vi "Get EasyXML Data Type.vi"(8 "error in":errorcluster, 10 "LabVIEW Data":variant) -> (0 "error out":errorcluster, 2 "EasyXML Type":T1=enum."Cluster")   [LabVIEW 2013]
uses:
  Type Defs/Formatting Data Type -- Enum.ctl
  <userlib>/_OpenG.lib/lvdata/lvdata.llb/Type Descriptor Enumeration__ogtk.ctl
  JKI Reuse Candidates/Is an Error (error cluster)__JKI Error Handling.vi
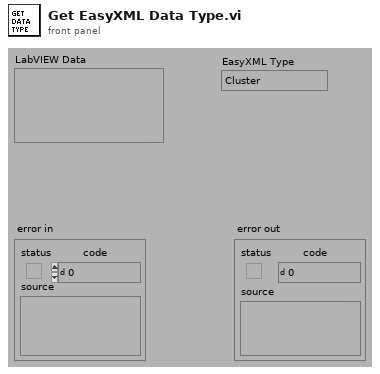
[diagram p1: front panel]
types:
  T1 = typedef "Formatting Data Type -- Enum.ctl" = enum16{"<unknown>", "Cluster", "Array", "String", "Path", "Boolean", "Time Stamp", "Enum", "Numeric - EXT", "Numeric - DBL", "Numeric - SGL", "Numeric - I64", "Numeric - I32", "Numeric - I16", "Numeric - I8", "Numeric - U64", "Numeric - U32", "Numeric - U16", "Numeric - U8", "Numeric - CXT", "Numeric - CDB", "Numeric - CSG", "VISA Resource"}
  T2 = typedef "Type Descriptor Enumeration__ogtk.ctl" = enum8{"<Null>", "I8", "I16", "I32", "I64", "U8", "U16", "U32", "U64", "SGL", "DBL", "EXT", "CSG", "CDB", "CXT", "0x0F", "0x10", "0x11", "0x12", "0x13", "0x14", "Enum U8", "Enum U16", "Enum U32", "Enum U64", "SGL PQ", "DBL PQ", "EXT PQ", "CSG PQ", "CDB PQ", "CXT PQ", "0x1F", "0x20", "Boolean", "0x22", "0x23", "0x24", "0x25", "0x26", "0x27", "0x28", "0x29", "0x2A", "0x2B", "0x2C", "0x2D", "0x2E", "0x2F", "String", "0x31", "Path", "Pict", "0x34", "0x35", "0x36", "DAQ", "0x38", "0x39", "0x3A", "0x3B", "0x3C", "0x3D", "0x3E", "0x3F", "Array", "0x41", "0x42", "0x43", "0x44", "0x45", "0x46", "0x47", "0x48", "0x49", "0x4A", "0x4B", "0x4C", "0x4D", "0x4E", "0x4F", "Cluster", "0x51", "0x52", "Variant", "Waveform", "0x55", "0x56", "0x57", "0x58", "0x59", "0x5A", "0x5B", "0x5C", "0x5D", "0x5E", "0x5F", "0x60", "0x61", "0x62", "0x63", "0x64", "0x65", "0x66", "0x67", "0x68", "0x69", "0x6A", "0x6B", "0x6C", "0x6D", "0x6E", "0x6F", "Refnum"}
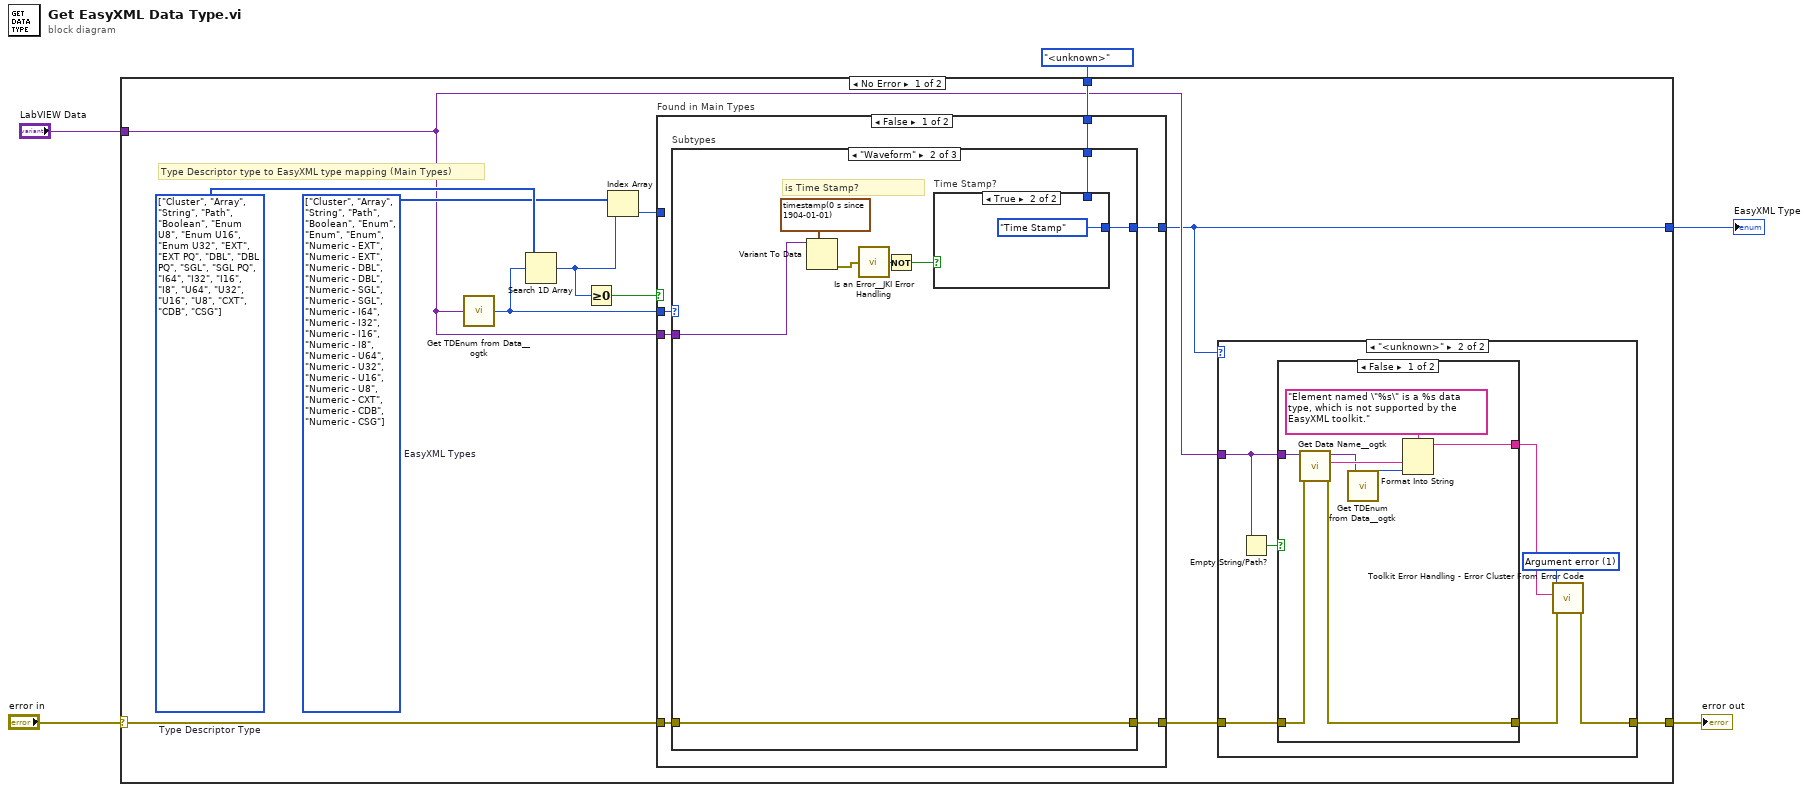
[diagram p0: block diagram]
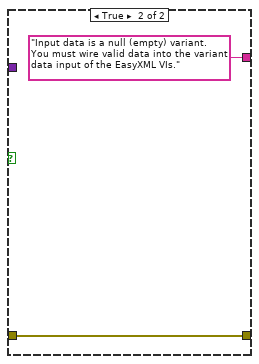
[diagram p3: hidden frame]
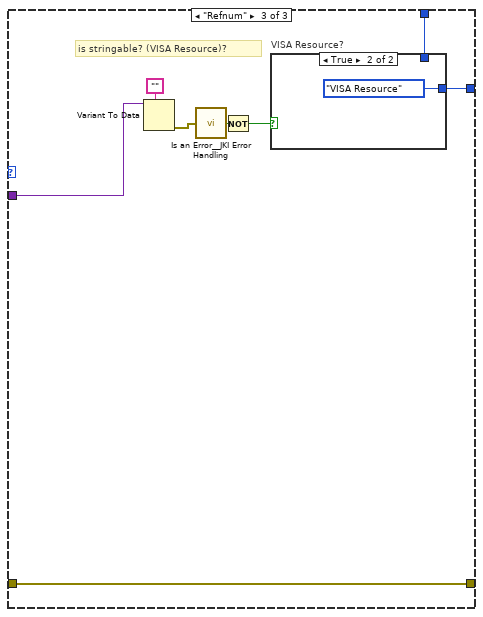
[diagram p6: hidden frame]
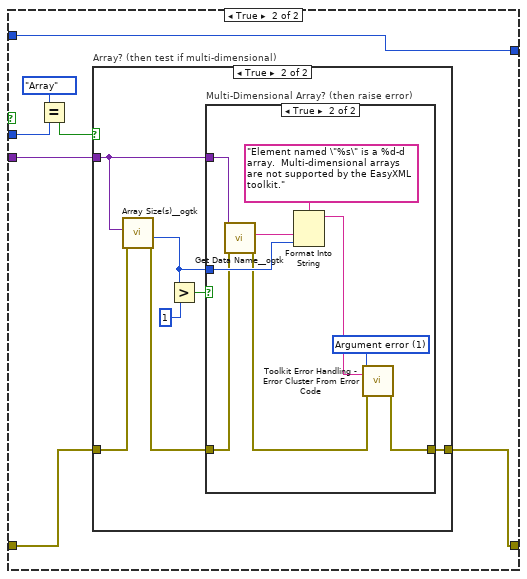
[diagram p8: hidden frame]
diagram:
  n1 = case shown="No Error" "error in" {
    selector: "error in" -> [w10 w89]
    tunnel: [w6 w90] -> w5
    tunnel: "LabVIEW Data" -> [w7 _]
    tunnel: Formatting_Data_Type_--_Enum."<unknown>" ("EasyXML Type") -> [w11 w90]
    tunnel: [w9 w89] -> w1
    frame No Error {
      w16 = T1[] [enum."Cluster", enum."Array", enum."String", enum."Path", enum."Boolean", enum."Enum", enum."Enum", enum."Enum", enum."Numeric - EXT", enum."Numeric - EXT", enum."Numeric - DBL", enum."Numeric - DBL", enum."Numeric - SGL", enum."Numeric - SGL", enum."Numeric - I64", enum."Numeric - I32", enum."Numeric - I16", enum."Numeric - I8", enum."Numeric - U64", enum."Numeric - U32", enum."Numeric - U16", enum."Numeric - U8", enum."Numeric - CXT", enum."Numeric - CDB", enum."Numeric - CSG"] items=["<unknown>", "Cluster", "Array", "String", "Path", "Boolean", "Time Stamp", "Enum", "Numeric - EXT", "Numeric - DBL", "Numeric - SGL", "Numeric - I64", "Numeric - I32", "Numeric - I16", "Numeric - I8", "Numeric - U64", "Numeric - U32", "Numeric - U16", "Numeric - U8", "Numeric - CXT", "Numeric - CDB", "Numeric - CSG", "VISA Resource"]  # EasyXML Types
      w17 = T2[] [enum."Cluster", enum."Array", enum."String", enum."Path", enum."Boolean", enum."Enum U8", enum."Enum U16", enum."Enum U32", enum."EXT", enum."EXT PQ", enum."DBL", enum."DBL PQ", enum."SGL", enum."SGL PQ", enum."I64", enum."I32", enum."I16", enum."I8", enum."U64", enum."U32", enum."U16", enum."U8", enum."CXT", enum."CDB", enum."CSG"] items=["<Null>", "I8", "I16", "I32", "I64", "U8", "U16", "U32", "U64", "SGL", "DBL", "EXT", "CSG", "CDB", "CXT", "0x0F", "0x10", "0x11", "0x12", "0x13", "0x14", "Enum U8", "Enum U16", "Enum U32", "Enum U64", "SGL PQ", "DBL PQ", "EXT PQ", "CSG PQ", "CDB PQ", "CXT PQ", "0x1F", "0x20", "Boolean", "0x22", "0x23", "0x24", "0x25", "0x26", "0x27", "0x28", "0x29", "0x2A", "0x2B", "0x2C", "0x2D", "0x2E", "0x2F", "String", "0x31", "Path", "Pict", "0x34", "0x35", "0x36", "DAQ", "0x38", "0x39", "0x3A", "0x3B", "0x3C", "0x3D", "0x3E", "0x3F", "Array", "0x41", "0x42", "0x43", "0x44", "0x45", "0x46", "0x47", "0x48", "0x49", "0x4A", "0x4B", "0x4C", "0x4D", "0x4E", "0x4F", "Cluster", "0x51", "0x52", "Variant", "Waveform", "0x55", "0x56", "0x57", "0x58", "0x59", "0x5A", "0x5B", "0x5C", "0x5D", "0x5E", "0x5F", "0x60", "0x61", "0x62", "0x63", "0x64", "0x65", "0x66", "0x67", "0x68", "0x69", "0x6A", "0x6B", "0x6C", "0x6D", "0x6E", "0x6F", "Refnum"]  # Type Descriptor Type
      # "Type Descriptor type to EasyXML type mapping (Main Types)"
      n2 = call <userlib>:"Get TDEnum from Data__ogtk.vi"("Data"=w7) -> ("Type Descriptor Enumeration"=w12:T2)  [unwired: 4 in]
      n3 = Search 1D Array(1D array=w17, element=w12) -> (index of element=w15:i32)  [unwired: 1 in]
      n4 = Greater Or Equal To 0?(x=w15) -> (x >= 0?=w14:bool)
      n5 = Index Array(array=w16, index=w15) -> (element=w13:T1)
      n6 = case "Found in Main Types" shown="False" w14 {
        tunnel: w13 -> [_ w70]
        tunnel: w12 -> [w41 w65]
        tunnel: [w39 w70] -> w6
        tunnel: w7 -> [w40 w67]
        tunnel: w11 -> [w38 _]
        tunnel: [w37 w68] -> w8
        tunnel: w10 -> [w36 w69]
        frame False {
          n7 = case "Subtypes" shown="\"Waveform\"" w41 {
            tunnel: w40 -> [_ w50 w61]
            tunnel: [w43 w47 w58] -> w39
            tunnel: w38 -> [w43 w46 w57]
            tunnel: [w42 w44 w55] -> w37
            tunnel: w36 -> [w42 w44 w55]
            frame Default {
            }
            frame "Waveform" {
              # "is Time Stamp?"
              n8 = Variant To Data(type=timestamp(0 s since 1904-01-01), Variant=w50) -> (error out=w49:errorcluster)  [unwired: 1 in, 1 out]
              n9 = call-poly "Is an Error__JKI Error Handling.vi"("error in"=w49) -> ("error?"=w48:bool)  [unwired: 8 in]
              n10 = Not(x=w48) -> (.not. x?=w45:bool)
              n11 = case "Time Stamp?" shown="True" w45 {
                tunnel: [w52 Formatting_Data_Type_--_Enum."Time Stamp" ("EasyXML Type")] -> w47
                tunnel: w46 -> [w52 _]
                frame False {
                }
                frame True {
                }
              }
            }
            frame "Refnum" {
              # "is stringable? (VISA Resource)?"
              n12 = Variant To Data(type="", Variant=w61) -> (error out=w60:errorcluster)  [unwired: 1 in, 1 out]
              n13 = call-poly "Is an Error__JKI Error Handling.vi"("error in"=w60) -> ("error?"=w59:bool)  [unwired: 8 in]
              n14 = Not(x=w59) -> (.not. x?=w56:bool)
              n15 = case "VISA Resource?" shown="True" w56 {
                tunnel: [w62 Formatting_Data_Type_--_Enum."VISA Resource" ("EasyXML Type")] -> w58
                tunnel: w57 -> [w62 _]
                frame False {
                }
                frame True {
                }
              }
            }
          }
        }
        frame True {
          n16 = Equal?(x=Type_Descriptor_Enumeration__ogtk."Array" ("Type Descriptor Enumeration"), y=w65) -> (x = y?=w64:bool)
          n17 = case "Array? (then test if multi-dimensional)" shown="True" w64 {
            tunnel: [w71 w75] -> w68
            tunnel: w69 -> [w71 w78]
            tunnel: w67 -> [_ w73]
            frame False {
            }
            frame True {
              n18 = call <userlib>:"Array Size(s)__ogtk.vi"("error in (no error)"=w78, "Array"=w73) -> ("error out"=w76:errorcluster, "N dims"=w72:u32)  [unwired: 7 in, 1 out]
              n19 = Greater?(x=w72, y=u32 1) -> (0:w74:bool)
              n20 = case "Multi-Dimensional Array? (then raise error)" shown="True" w74 {
                tunnel: [w79 w82] -> w75
                tunnel: w76 -> [w79 w81]
                tunnel: w73 -> [_ w88]
                tunnel: w72 -> [_ w85]
                frame False {
                }
                frame True {
                  w84 = 1 items=["No error", "Argument error", "Memory is full", "Out of zone", "End of file", "File already open", "Generic file I/O error", "File not found", "File permission error", "Disk is full", "Duplicate path", "Too many files open", "System feature not enabled", "Resource file not found", "Cannot add resource", "Resource not found", "Image not found", "Image memory error", "Pen does not exist", "Config type invalid", "Config token not found", "Config parse error", "Config memory error", "Bad external code format", "Bad external code offset", "External code not present", "Null window", "Destroy window error", "Null menu", "Print aborted", "Bad print record", "Print driver error", "Windows error during printing", "Memory error during printing", "Print dialog error", "Generic print error", "Invalid device refnum", "Device not found", "Device parameter error", "Device unit error", "Cannot open device", "Device call aborted", "Generic error", "Cancelled by user", "Object ID too low", "Object ID too high", "Object not in heap", "Unknown heap", "Unknown object (invalid DefProc)", "Unknown object (DefProc not in table)", "Message out of range", "Invalid (null) method", "Unknown message", "Manager call not supported", "Bad address", "Network operation in progress", "Network operation timed out", "Connection is busy", "Network attribute not supported", "Network error", "Address in use", "System out of memory", "Connection aborted", "Connection refused", "Not connected", "Already connected", "Connection closed", "Initialization error (interapplication manager)", "Bad occurrence", "Wait on unbound occurrence handler", "Occurrence queue overflow", "Datalog type conflict", "Unused", "Unrecognized type (interapplication manager)", "Memory corrupt", "Failed to make temporary DLL", "Old CIN version", "Drag socket not found", "Failed to load drop-object", "Failed to register OLE object", "Failed to release OLE object", "Format specifier type mismatch", "Unknown format specifier", "Too few format specifiers", "Too many format specifiers", "Scan failed", "Newer CIN version", "Error converting to variant", "Runtime menu error", "Password tampered", "Variant attribute not found", "Incompatible variant data type", "Event data is not available", "Event Store is not present", "Occurrence is not found", "Event Queue is not created", "Event info is not available", "Refnum passed is NULL", "Error retrieving Class GUID", "Error retrieving CoClass GUID", "Error retrieving TypeLib GUID.", "Bad built application magic bytes.", "Specific driver is different from the specific driver associated with the Logical Name.", "There is no session opened to the class driver.", "Max Error", "MAX - Error with config objects", "MAX - Error loading configuration", "MAX - Group not supported"]
                  n21 = call <userlib>:"Get Data Name__ogtk.vi"("error in (no error)"=w81, "Data"=w88) -> ("error out"=w80:errorcluster, "Data Name"=w87:string)  [unwired: 7 in, 1 out]
                  n22 = Format Into String(format string="Element named \"%s\" is a %d-d array.  Multi-dimensional arrays are not supported by the EasyXML toolkit." ("Format String"), w87, w85) -> (resulting string=w83:string)  [unwired: 2 in, 1 out]
                  n23 = call "Toolkit Error Handling - Error Cluster From Error Code.vi"("error in"=w80, "error message (\"\")"=w83, "error code (0)"=w84) -> ("error out"=w82:errorcluster)  [unwired: 6 in]
                }
              }
            }
          }
        }
      }
      n24 = case shown="\"<unknown>\"" w6 {
        tunnel: [w18 w21] -> w9
        tunnel: w8 -> [w18 w22]
        tunnel: w7 -> [_ w19]
        frame Default {
        }
        frame "<unknown>" {
          w25 = 1 items=["No error", "Argument error", "Memory is full", "Out of zone", "End of file", "File already open", "Generic file I/O error", "File not found", "File permission error", "Disk is full", "Duplicate path", "Too many files open", "System feature not enabled", "Resource file not found", "Cannot add resource", "Resource not found", "Image not found", "Image memory error", "Pen does not exist", "Config type invalid", "Config token not found", "Config parse error", "Config memory error", "Bad external code format", "Bad external code offset", "External code not present", "Null window", "Destroy window error", "Null menu", "Print aborted", "Bad print record", "Print driver error", "Windows error during printing", "Memory error during printing", "Print dialog error", "Generic print error", "Invalid device refnum", "Device not found", "Device parameter error", "Device unit error", "Cannot open device", "Device call aborted", "Generic error", "Cancelled by user", "Object ID too low", "Object ID too high", "Object not in heap", "Unknown heap", "Unknown object (invalid DefProc)", "Unknown object (DefProc not in table)", "Message out of range", "Invalid (null) method", "Unknown message", "Manager call not supported", "Bad address", "Network operation in progress", "Network operation timed out", "Connection is busy", "Network attribute not supported", "Network error", "Address in use", "System out of memory", "Connection aborted", "Connection refused", "Not connected", "Already connected", "Connection closed", "Initialization error (interapplication manager)", "Bad occurrence", "Wait on unbound occurrence handler", "Occurrence queue overflow", "Datalog type conflict", "Unused", "Unrecognized type (interapplication manager)", "Memory corrupt", "Failed to make temporary DLL", "Old CIN version", "Drag socket not found", "Failed to load drop-object", "Failed to register OLE object", "Failed to release OLE object", "Format specifier type mismatch", "Unknown format specifier", "Too few format specifiers", "Too many format specifiers", "Scan failed", "Newer CIN version", "Error converting to variant", "Runtime menu error", "Password tampered", "Variant attribute not found", "Incompatible variant data type", "Event data is not available", "Event Store is not present", "Occurrence is not found", "Event Queue is not created", "Event info is not available", "Refnum passed is NULL", "Error retrieving Class GUID", "Error retrieving CoClass GUID", "Error retrieving TypeLib GUID.", "Bad built application magic bytes.", "Specific driver is different from the specific driver associated with the Logical Name.", "There is no session opened to the class driver.", "Max Error", "MAX - Error with config objects", "MAX - Error loading configuration", "MAX - Group not supported"]
          n25 = Empty String/Path?(string/path=w19) -> (empty?=w20:bool)
          n26 = case shown="False" w20 {
            tunnel: [w32 "Input data is a null (empty) variant.  You must wire valid data into the variant data input of the EasyXML VIs." ("Format String")] -> w24
            tunnel: [w31 w35] -> w23
            tunnel: w22 -> [w29 w35]
            tunnel: w19 -> [w27 _]
            frame False {
              n27 = call <userlib>:"Get Data Name__ogtk.vi"("error in (no error)"=w29, "Data"=w27) -> ("error out"=w31:errorcluster, "Data Name"=w30:string, "Data dup"=w26:variant)  [unwired: 7 in]
              n28 = call <userlib>:"Get TDEnum from Data__ogtk.vi"("Data"=w26) -> ("Type Descriptor Enumeration"=w28:T2)  [unwired: 4 in]
              n29 = Format Into String(format string="Element named \"%s\" is a %s data type, which is not supported by the EasyXML toolkit." ("Format String"), w30, w28) -> (resulting string=w32:string)  [unwired: 2 in, 1 out]
            }
            frame True {
            }
          }
          n30 = call "Toolkit Error Handling - Error Cluster From Error Code.vi"("error in"=w23, "error message (\"\")"=w24, "error code (0)"=w25) -> ("error out"=w21:errorcluster)  [unwired: 6 in]
        }
      }
    }
    frame Error {
    }
  }
  "EasyXML Type" <- w5
  "error out" <- w1
